vi "Create.vi"(7 "options":T13, 8 "error in (no error)":errorcluster, 11 "Device Item Ref":T18=18446744073709551615 format="%.0x") -> (0 "error out":errorcluster, 2 "framework configuration":T1, 3 "VeriStand Framework":refnum<class "VeriStand DSF.lvclass">)   [LabVIEW 2017, in "DSF Engine.lvlib" / "VeriStand DSF.lvclass"]
uses:
  VeriStand DSF.lvclass
  <vilib>/NI Veristand/Custom Device API/Custom Device Item Ref.ctl
  DSF Core.lvlibp/Classes/Framework/Framework Options.ctl
  DSF Core.lvlibp/Typedefs/DSF FIFO Options.ctl
  DSF Core.lvlibp/Classes/Thread/DSF Thread Options.ctl
  DSF Core.lvlibp/Typedefs/DSF Plugin Options.ctl
  DSF Core.lvlibp/Typedefs/DSF Performance Options.ctl
  DSF Core.lvlibp/Typedefs/DSF Engine Framework Configuration.ctl
  DSF Core.lvlibp/Typedefs/DSF Engine Plugin Configuration.ctl
  DSF Core.lvlibp/Typedefs/DSF Timing Info.ctl
  DSF Core.lvlibp/Typedefs/DSF Engine Plugin Thread Configuration.ctl
  DSF Core.lvlibp/Typedefs/DSF Settings Info.ctl
  DSF Core.lvlibp/Typedefs/DSF Engine Transfer Group Configuration.ctl
  DSF Core.lvlibp/Typedefs/DSF Direction.ctl
  DSF Core.lvlibp/Typedefs/DSF Engine Transfer Configuration.ctl
  DSF Core.lvlibp/Typedefs/DSF Byte Order.ctl
  DSF Core.lvlibp/Typedefs/DSF Engine Channel Configuration.ctl
  DSF Core.lvlibp/Typedefs/DSF Data Type.ctl
  DSF Core.lvlibp/Typedefs/DSF Timeout Behavior.ctl
  VeriStand DSF.lvclass/VeriStand DSF.ctl
  DSF Core.lvlibp/Classes/Configuration/Configuration Session.lvclass
  Shared/DSF Shared.lvlib
  <vilib>/NI Veristand/Custom Device API/Custom Device API.lvlib
  DSF Core.lvlibp/Classes/Framework/Framework.lvclass
  DSF Core.lvlibp
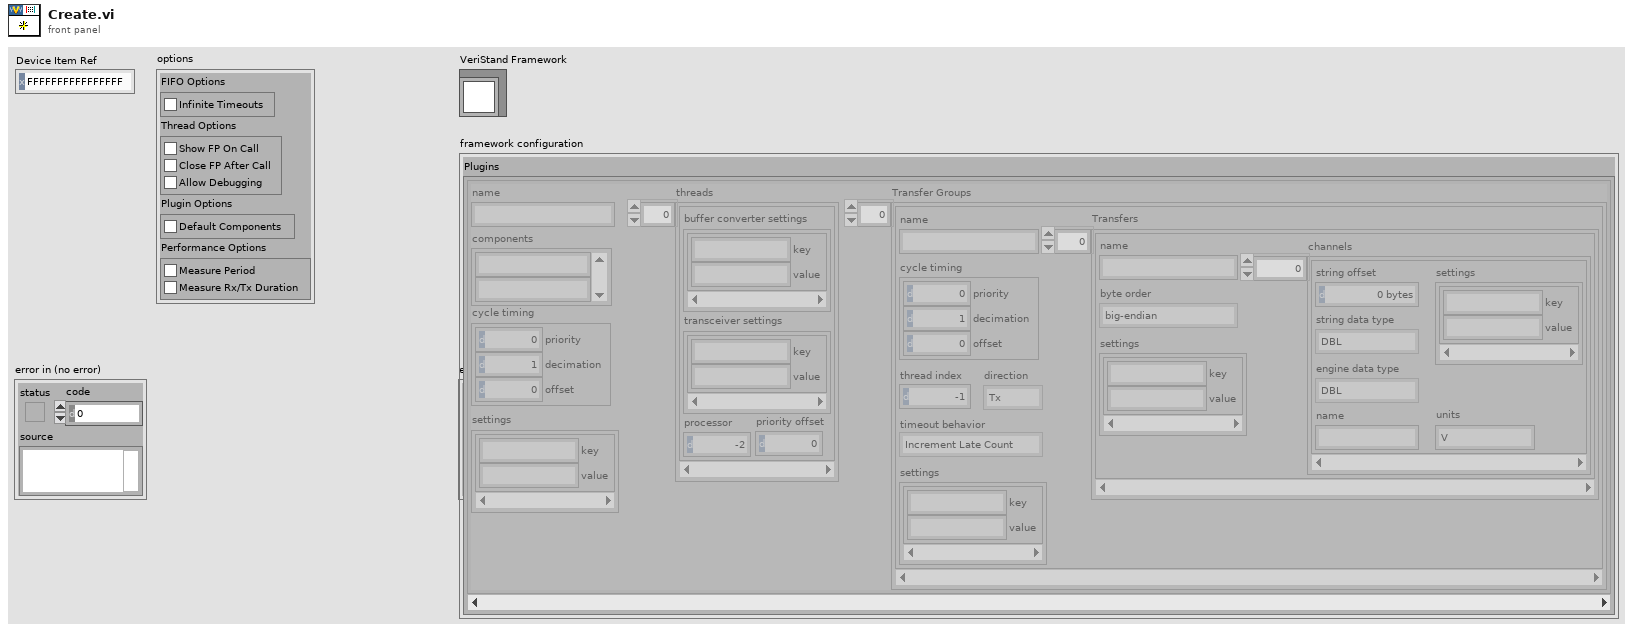
[diagram p1: front panel]
types:
  T1 = typedef "DSF Core.lvlibp/DSF Engine Framework Configuration.ctl" = cluster{"Plugins":T2[]}
  T2 = typedef "DSF Core.lvlibp/DSF Engine Plugin Configuration.ctl" = cluster{"name":string, "components":string[], "cycle timing":T3, "threads":T4[], "Transfer Groups":T6[], "settings":T5}
  T3 = typedef "DSF Core.lvlibp/DSF Timing Info.ctl" = cluster{"priority":u64, "decimation":u64, "offset":u64}
  T4 = typedef "DSF Core.lvlibp/DSF Engine Plugin Thread Configuration.ctl" = cluster{"buffer converter settings":T5, "transceiver settings":T5, "processor":i32, "priority offset":i16}
  T5 = typedef "DSF Core.lvlibp/DSF Settings Info.ctl" = cluster{"key":string, "value":string}[]
  T6 = typedef "DSF Core.lvlibp/DSF Engine Transfer Group Configuration.ctl" = cluster{"name":string, "direction":T7, "cycle timing":T3, "thread index":i32, "settings":T5, "Transfers":T8[], "timeout behavior":T12}
  T7 = typedef "DSF Core.lvlibp/DSF Direction.ctl" = enum8{"Tx", "Rx"}
  T8 = typedef "DSF Core.lvlibp/DSF Engine Transfer Configuration.ctl" = cluster{"name":string, "byte order":T9, "settings":T5, "channels":T10[]}
  T9 = typedef "DSF Core.lvlibp/DSF Byte Order.ctl" = enum8{"big-endian", "little-endian"}
  T10 = typedef "DSF Core.lvlibp/DSF Engine Channel Configuration.ctl" = cluster{"string offset":u64, "string data type":T11, "engine data type":T11, "name":string, "settings":T5, "units":string}
  T11 = typedef "DSF Core.lvlibp/DSF Data Type.ctl" = enum8{"Bool", "SGL", "DBL", "I8", "I16", "I32", "I64", "U8", "U16", "U32", "U64"}
  T12 = typedef "DSF Core.lvlibp/DSF Timeout Behavior.ctl" = enum8{"Increment Late Count", "Throw Error"}
  T13 = typedef "DSF Core.lvlibp/Framework.lvclass/Framework Options.ctl" = cluster{"FIFO Options":T14, "Thread Options":T15, "Plugin Options":T16, "Performance Options":T17}
  T14 = typedef "DSF Core.lvlibp/DSF FIFO Options.ctl" = cluster{"Infinite Timeouts":bool}
  T15 = typedef "DSF Core.lvlibp/DSF Thread Options.ctl" = cluster{"Show FP On Call":bool, "Close FP After Call":bool, "Allow Debugging":bool}
  T16 = typedef "DSF Core.lvlibp/DSF Plugin Options.ctl" = cluster{"Default Components":bool}
  T17 = typedef "DSF Core.lvlibp/DSF Performance Options.ctl" = cluster{"Measure Period":bool, "Measure Rx/Tx Duration":bool}
  T18 = typedef "Custom Device API.lvlib/Custom Device Item Ref.ctl" = u64
  T19 = enum16{"open", "replace", "create", "open or create", "replace or create", "replace or create with confirmation"}
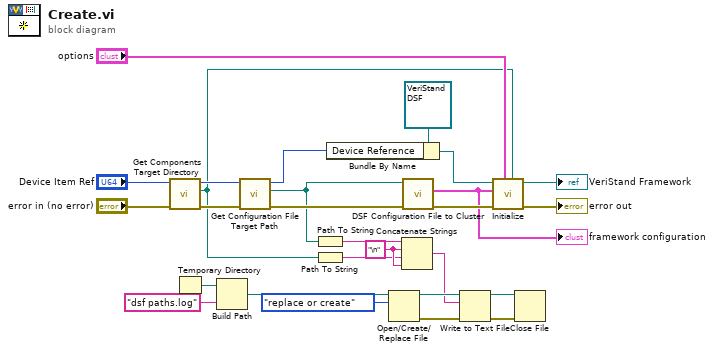
[diagram p0: block diagram]
diagram:
  w12 = "\n" ("string")
  n1 = call "Get Components Target Directory.vi"("error in (no error)"="error in (no error)", "Item Ref in"="Device Item Ref") -> ("error out"=w6:errorcluster, "components target directory"=w1:path, "Item Ref out"=w5:T18)  [unwired: 7 in]
  n2 = Temporary Directory() -> (w9:path)
  n3 = Build Path(base path=w9, name or relative path="dsf paths.log" ("file path (use dialog)")) -> (appended path=w7:path)
  n4 = call "Get Configuration File Target Path.vi"("error in (no error)"=w6, "Item Ref in"=w5) -> ("error out"=w3:errorcluster, "configuration target path"=w2:path, "Item Ref out"=w4:T18)  [unwired: 7 in]
  n5 = Path To String(path=w2) -> (string=w13:string)
  n6 = Path To String(path=w1) -> (string=w11:string)
  n7 = Bundle By Name(cluster=refnum<class "VeriStand DSF.lvclass"> refnum ("VeriStand Data Sharing Framework out"), "Device Reference"=w4) -> (w24:refnum<class "VeriStand DSF.lvclass">)
  n8 = Open/Create/Replace File(file path (use dialog)=w7, operation (0:open)=T19."replace or create") -> (refnum out=w20:refnum<file>, error out=w21:errorcluster)  [unwired: 4 in, 1 out]
  n9 = Concatenate Strings(w13, w12, w11, w12) -> (w10:string)
  n10 = call "DSF Configuration File to Cluster.vi"("error in (no error)"=w3, "dsf configuration file path"=w2) -> ("error out"=w25:errorcluster, "framework configuration out"=w16:T1)  [unwired: 7 in, 1 out]
  "framework configuration" <- w16
  n11 = Write to Text File(file (use dialog)=w20, text=w10, error in=w21) -> (refnum out=w18:refnum<file>, error out=w19:errorcluster)  [unwired: 1 in, 1 out]
  n12 = call-dynamic "Initialize.vi"("components directory"=w1, "options"="options", "error in (no error)"=w25, "framework configuration"=w16, "VeriStand Data Sharing Framework in"=w24) -> ("error out"=→"error out":errorcluster, "VeriStand Data Sharing Framework out"=→"VeriStand Framework":refnum<class "VeriStand DSF.lvclass">)  [unwired: 5 in]
  n13 = Close File(refnum=w18, error in=w19) -> ()  [unwired: 2 out]
